vi "extract jitter data.vi"() -> ()   [LabVIEW 2009]
uses:
  <vilib>/Utility/file.llb/Read From Spreadsheet File (I64).vi
panel:
  out "total time elapsed":string
  out "Waveform Graph":i64[](graph)
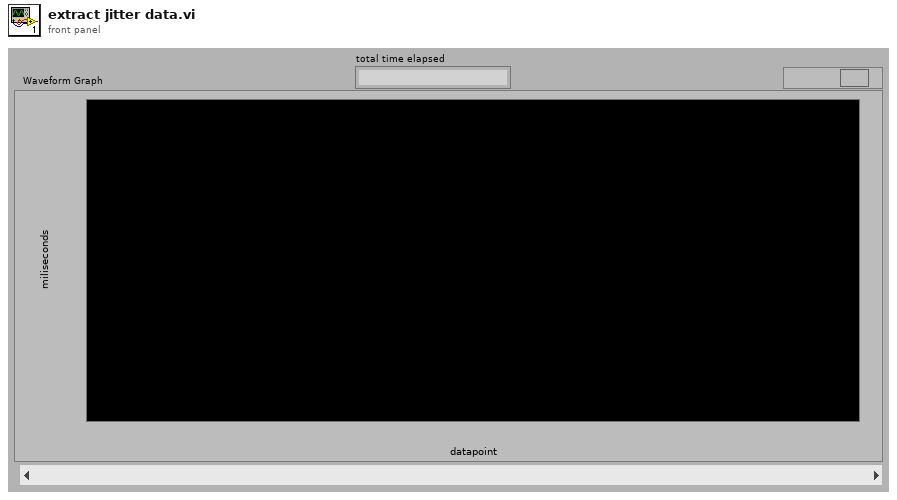
[diagram p1: front panel]
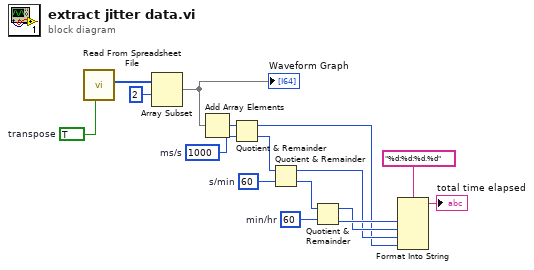
[diagram p0: block diagram]
diagram:
  w10 = i64 60  # min/hr
  w12 = i64 60  # s/min
  w14 = i64 1000  # ms/s
  w16 = TRUE  # transpose
  n1 = call-poly <vilib>:"Read From Spreadsheet File.vi"("transpose (no:F)"=w16) -> ("first row"=w1:i64[])  [unwired: 6 in, 4 out]
  n2 = Array Subset(array=w1, index=2) -> (w9:i64[])  [unwired: 1 in]
  "Waveform Graph" <- w9
  n3 = Add Array Elements(numeric array=w9) -> (sum=w15:i64)
  n4 = Quotient & Remainder(x=w15, y=w14) -> (x-y*floor(x/y)=w4:i64, floor(x/y)=w13:i64)
  n5 = Quotient & Remainder(x=w13, y=w12) -> (x-y*floor(x/y)=w5:i64, floor(x/y)=w11:i64)
  n6 = Quotient & Remainder(x=w11, y=w10) -> (x-y*floor(x/y)=w6:i64, floor(x/y)=w7:i64)
  n7 = Format Into String(format string="%d:%d:%d.%d", w7, w6, w5, w4) -> (resulting string=→"total time elapsed":string)  [unwired: 2 in, 1 out]
